vi "RC_Generate_Condition_text.vi"(8 "error in (no error)":errorcluster, 10 "Calibration parameters":T1={"Timing calibration sw/hw"=1.0, "True FPS"=80.0, "True frame time, s"=0.0125, "Disp. calibration info"=[]} {"True frame time, s" format="%.10g"; "Disp. calibration info"."Speed, µl per ms" format="%.3g"; "True FPS" format="%.10g"; "Timing calibration sw/hw" format="%.10g"}, 11 "Condition in":refnum<class "Reward_Condition.lvclass">) -> (0 "error out":errorcluster, 2 "Validity criteria":string[](array[string]), 3 "SubCondition":string[](array[string]))   [LabVIEW 2018, in "Tracker.lvlib" / "Reward_Condition.lvclass"]
uses:
  Reward_Condition.lvclass
  Controls/CTL_Calibration_parameters.ctl
  Controls/CTL_Dispenser_calibration_info.ctl
  Reward_SubCondition/Reward_SubCondition.lvclass
  Reward_Condition.lvclass/Reward_Condition.ctl
  Tracker.lvlib
panel:
  in  "Dev mode?":bool
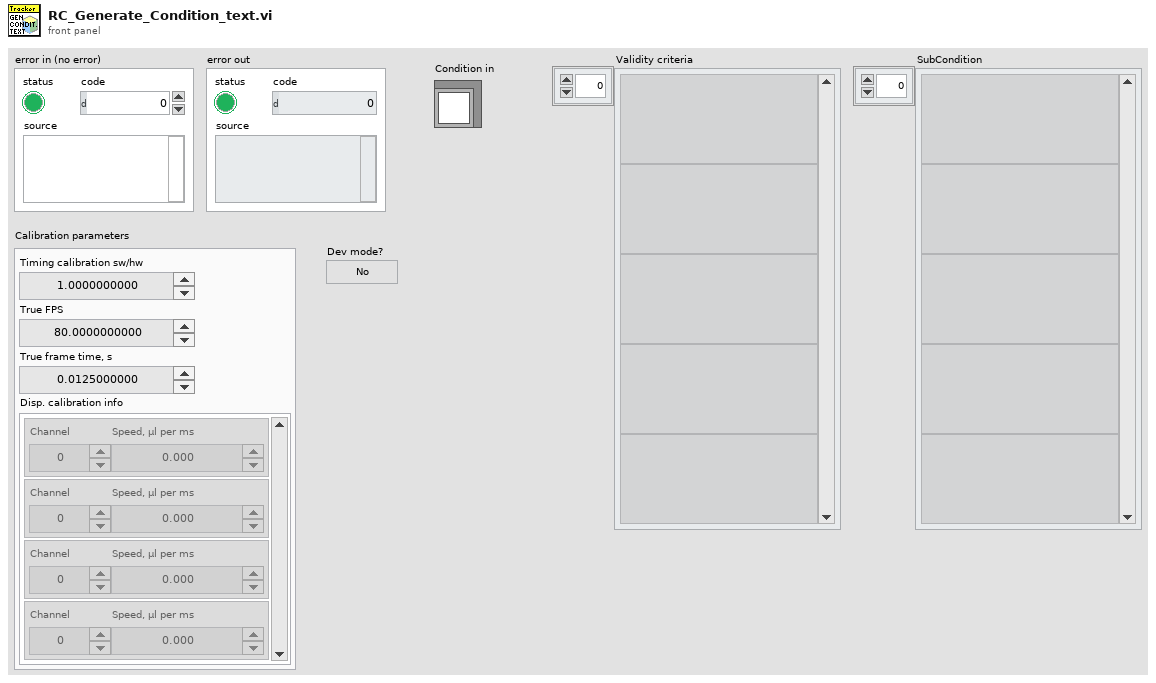
[diagram p1: front panel]
types:
  T1 = typedef "Tracker.lvlib/CTL_Calibration_parameters.ctl" = cluster{"Timing calibration sw/hw":dbl, "True FPS":dbl, "True frame time, s":dbl, "Disp. calibration info":T2}
  T2 = typedef "Tracker.lvlib/CTL_Dispenser_calibration_info.ctl" = cluster{"Channel":u8, "Speed, µl per ms":dbl}[]
  T3 = cluster{"Enabled":bool, "Type":enum16{"Angle to wall", "Speed", "Zone"}, "Comparison type":enum16{"Less", "Less or Equal", "Equal", "Greater or Equal", "Greater", "Not Equal"}, "Comparison value":dbl, "Validity check Enabled":bool, "Criteria to check":enum16{"Running bout, sec", "Running bout, m"}, "Has been True for, units":dbl}
  T4 = enum16{"None", "TTL pulse", "TTL trigger", "Air puff", "Liquid reward"}
  T5 = enum16{"None", "Port 1", "Port 2", "Port 3", "Port 4"}
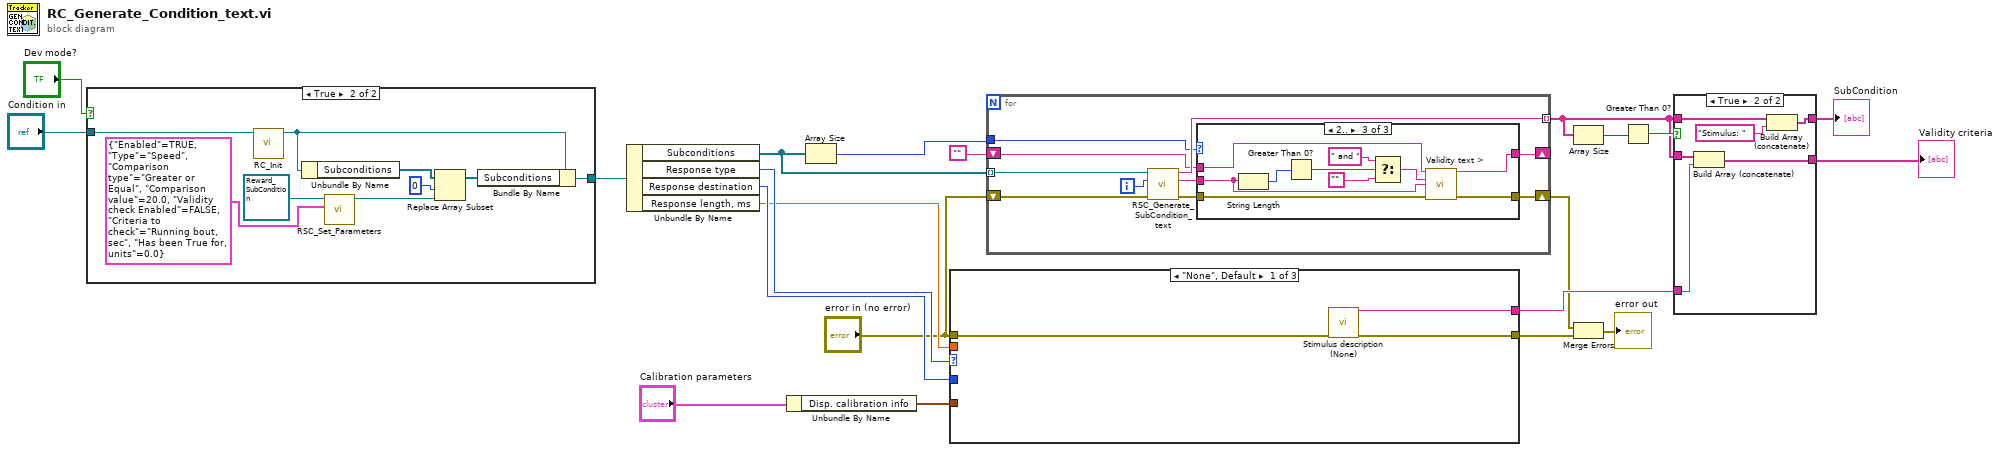
[diagram p0: block diagram]
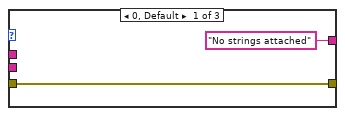
[diagram p3: hidden frame]
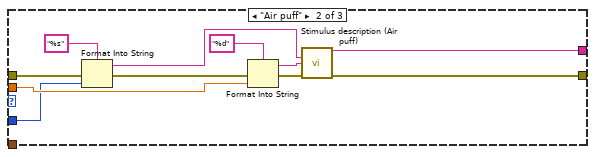
[diagram p6: hidden frame]
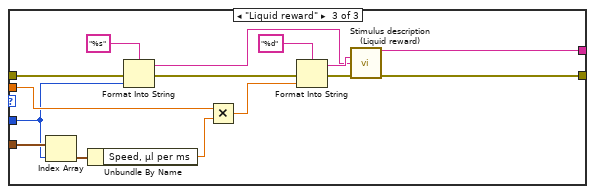
[diagram p7: hidden frame]
diagram:
  n1 = case shown="True" "Dev mode?" {
    tunnel: "Condition in" -> [w22 w31]
    tunnel: [w22 w23] -> w2
    frame False {
    }
    frame True {
      n2 = call "RC_Init.vi"("Reward_Condition in"=w31) -> ("Reward_Condition out"=w25:refnum<class "Reward_Condition.lvclass">)  [unwired: 9 in, 1 out]
      n3 = Unbundle By Name(w25) -> ("Subconditions"=w30:refnum<class "Reward_SubCondition.lvclass">[])
      n4 = call "RSC_Set_Parameters.vi"("Data to update"=T3 {"Enabled"=TRUE, "Type"=enum."Speed", "Comparison type"=enum."Greater or Equal", "Comparison value"=20.0, "Validity check Enabled"=FALSE, "Criteria to check"=enum."Running bout, sec", "Has been True for, units"=0.0}, "Reward_SubCondition in"=refnum<class "Reward_SubCondition.lvclass"> refnum ("new element/subarray")) -> ("Reward_SubCondition out"=w27:refnum<class "Reward_SubCondition.lvclass">)  [unwired: 8 in, 1 out]
      n5 = Replace Array Subset(array=w30, new element=w27, index=0) -> (w24:refnum<class "Reward_SubCondition.lvclass">[])
      n6 = Bundle By Name(cluster=w25, "Subconditions"=w24) -> (w23:refnum<class "Reward_Condition.lvclass">)
    }
  }
  n7 = Unbundle By Name(w2) -> ("Subconditions"=w6:refnum<class "Reward_SubCondition.lvclass">[], "Response type"=w12:T4, "Response destination"=w11:T5, "Response length, ms"=w10:dbl)
  n8 = Unbundle By Name("Calibration parameters") -> ("Disp. calibration info"=w13:T2)
  n9 = Array Size(array=w6) -> (size(s)=w7:i32)
  n10 = case shown="\"None\", Default" w12 {
    tunnel: "error in (no error)" -> [w34 w38 w49]
    tunnel: [w33 w45 w60] -> w20
    tunnel: [w32 w44 w59] -> w18
    tunnel: w11 -> [_ w35 w48]
    tunnel: w10 -> [_ w42 w57]
    tunnel: w13 -> [_ _ w54]
    frame "None", Default {
      n11 = call "Stimulus description (None)"("error in (no error)"=w34) -> ("Result"=w32:string, "error out"=w33:errorcluster)  [unwired: 13 in]
    }
    frame "Air puff" {
      n12 = Format Into String(format string="%s", error in=w38, w35) -> (resulting string=w36:string, error out=w37:errorcluster)  [unwired: 1 in]
      n13 = Format Into String(format string="%d", error in=w37, w42) -> (resulting string=w40:string, error out=w41:errorcluster)  [unwired: 1 in]
      n14 = call "Stimulus description (Air puff)"("port"=w36, "length"=w40, "error in (no error)"=w41) -> ("Result"=w44:string, "error out"=w45:errorcluster)  [unwired: 11 in]
    }
    frame "Liquid reward" {
      n15 = Index Array(array=w54, index=w48) -> (element=w53:cluster{"Channel":u8, "Speed, µl per ms":dbl})
      n16 = Unbundle By Name(w53) -> ("Speed, µl per ms"=w51:dbl)
      n17 = Format Into String(format string="%s", error in=w49, w48) -> (resulting string=w47:string, error out=w46:errorcluster)  [unwired: 1 in]
      n18 = Multiply(x=w57, y=w51) -> (x*y=w52:dbl)
      n19 = Format Into String(format string="%d", error in=w46, w52) -> (resulting string=w55:string, error out=w56:errorcluster)  [unwired: 1 in]
      n20 = call "Stimulus description (Liquid reward)"("amount"=w55, "port"=w47, "error in (no error)"=w56) -> ("Result"=w59:string, "error out"=w60:errorcluster)  [unwired: 11 in]
    }
  }
  n21 = for {
    tunnel: w6 -> [w69] mode=indexing
    tunnel: [w68] -> w4 mode=indexing
    shift-right: [w65] -> w8
    shift-left: "error in (no error)" -> [w70]
    tunnel: w7 -> [w63]
    shift-right: [w61] -> _
    shift-left: "" -> [w62]
    i -> [w64]
    n22 = call "RSC_Generate_SubCondition_text.vi"("error in (no error)"=w70, "SubCondition #"=w64, "Subcondition"=w69) -> ("error out"=w67:errorcluster, "Validity Criteria"=w66:string, "Condition Info"=w68:string)  [unwired: 6 in]
    n23 = case shown="2.." w63 {
      tunnel: w66 -> [_ w73 w75]
      tunnel: ["No strings attached" ("Result") w73 w84] -> w61
      tunnel: w67 -> [w71 w74 w83]
      tunnel: [w71 w74 w82] -> w65
      tunnel: w62 -> [_ _ w77]
      frame 0, Default {
      }
      frame 1 {
      }
      frame 2.. {
        n24 = String Length(string=w75) -> (length=w76:i32)
        n25 = Greater Than 0?(x=w76) -> (x > 0?=w81:bool)
        n26 = Select(t=" and ", s=w81, f="") -> (s? t:f=w78:string)
        n27 = call "Validity text >"("Beginning Text"=w77, "midtext"=w78, "endtext"=w75, "error in (no error)"=w83) -> ("Result"=w84:string, "error out"=w82:errorcluster)  [unwired: 10 in]
      }
    }
  }
  n28 = Array Size(array=w4) -> (size(s)=w17:i32)
  n29 = Merge Errors(w8, w20) -> (→"error out":errorcluster)
  n30 = Greater Than 0?(x=w17) -> (x > 0?=w16:bool)
  n31 = case shown="True" w16 {
    tunnel: [w86 w92] -> w19
    tunnel: w18 -> [_ w91]
    tunnel: w4 -> [w86 w90]
    tunnel: w4 -> [w85 w89]
    tunnel: [w85 w87] -> w15
    frame False {
    }
    frame True {
      n32 = Build Array (concatenate)(w90, w91) -> (w92:string[])
      n33 = Build Array (concatenate)(w89, "Stimulus: ") -> (w87:string[])
    }
  }
  "Validity criteria" <- w19
  "SubCondition" <- w15
